vi "Set Fetch Step Values.vi"(8 "error in (no error)":errorcluster, 11 "SPECAN_IQSLOT in":refnum<class "SPECAN_IQSLOT.lvclass">) -> (0 "error out":errorcluster, 2 "Step Out":refnum<k7>, 3 "SPECAN_IQSLOT out":refnum<class "SPECAN_IQSLOT.lvclass">)   [LabVIEW 2018, in "SPECAN_IQSLOT.lvlib" / "SPECAN_IQSLOT.lvclass"]
uses:
  SPECAN_IQSLOT.lvclass
  Plugins/Measurement Interface.lvlibp/Measurement Interface.lvclass
  C:/Sequence Automation/Plugins/Measurement Interface.lvlibp/Measurement Interface.lvclass
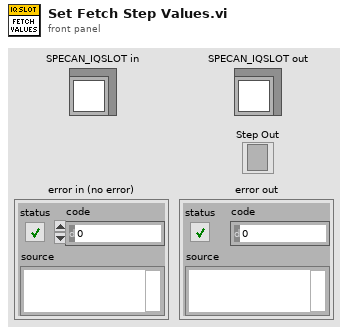
[diagram p1: front panel]
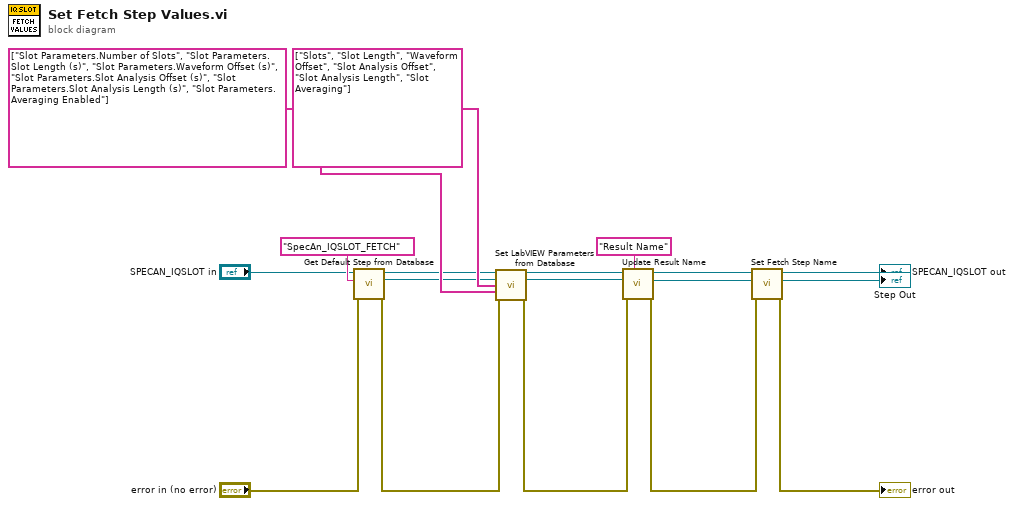
[diagram p0: block diagram]
diagram:
  n1 = call "Get Default Step from Database.vi"("error in (no error)"="error in (no error)", "Default Step"="SpecAn_IQSLOT_FETCH", "Measurement Interface in"="SPECAN_IQSLOT in") -> ("error out"=w13:errorcluster, "Cloned Step"=w12:refnum<k7>, "Measurement Interface out"=w11:refnum<class "SPECAN_IQSLOT.lvclass">)  [unwired: 6 in]
  n2 = call "Set LabVIEW Parameters from Database.vi"("Measurement Interface in"=w11, "Step In"=w12, "Dictionary Keys"=string[] ["Slots", "Slot Length", "Waveform Offset", "Slot Analysis Offset", "Slot Analysis Length", "Slot Averaging"] ("LabVIEW Parameter Mapping"), "LabVIEW Parameter Mapping"=string[] ["Slot Parameters.Number of Slots", "Slot Parameters.Slot Length (s)", "Slot Parameters.Waveform Offset (s)", "Slot Parameters.Slot Analysis Offset (s)", "Slot Parameters.Slot Analysis Length (s)", "Slot Parameters.Averaging Enabled"] ("Dictionary Keys"), "error in (no error)"=w13) -> ("Measurement Interface out"=w15:refnum<class "SPECAN_IQSLOT.lvclass">, "Step Out"=w16:refnum<k7>, "error out"=w14:errorcluster)  [unwired: 8 in]
  n3 = call-dynamic "Update Result Name.vi"("LabVIEW Result Name Parameter"="Result Name", "error in (no error)"=w14, "Step In"=w16, "SPECAN_IQSLOT in"=w15) -> ("error out"=w10:errorcluster, "Step Out"=w2:refnum<k7>, "SPECAN_IQSLOT out"=w4:refnum<class "SPECAN_IQSLOT.lvclass">)  [unwired: 5 in]
  n4 = call "Set Fetch Step Name.vi"("error in (no error)"=w10, "Step In"=w2, "SPECAN_IQSLOT in"=w4) -> ("error out"=→"error out":errorcluster, "Step Out"=→"Step Out":refnum<k7>, "SPECAN_IQSLOT out"=→"SPECAN_IQSLOT out":refnum<class "SPECAN_IQSLOT.lvclass">)  [unwired: 6 in]
